vi "p2.vi"() -> ()   [LabVIEW 2021, in "d22.lvlib"]
uses:
  d22.lvlib
  AOC/AOC.lvlib
panel:
  out "Total Instructions":i32
  out "Instruction":i32
  out "Vis":T1(graph)
  out "facing":enum16{"R", "D", "L", "U"}(ring)=enum."L"
  out "col":i32=43
  out "row":i32=133
  in  "Example":string="        ...#\n        .#..\n        #...\n        ....\n...#.......#\n........#...\n..#....#....\n..........#.\n        ...#....\n        .....#..\n        .#......\n        ......#.\n\n10R5L5R10L4R5L5"
  in  "Example":bool
  out "Answer":i32=133174
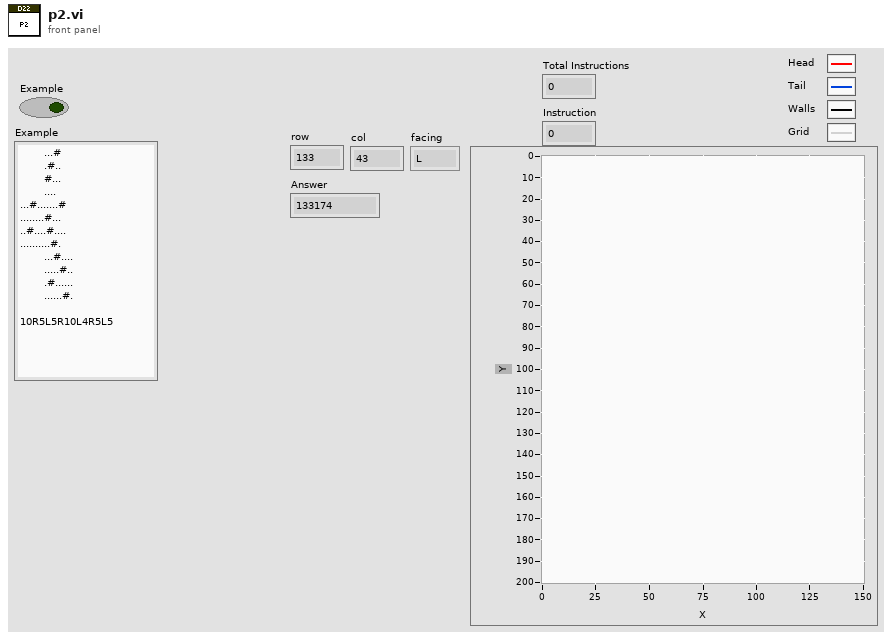
[diagram p1: front panel]
types:
  T1 = cluster{"index of element":i32[], "index of element":i32[]}[]
  T2 = cluster{"index of element":i32[], "index of element":i32[]}
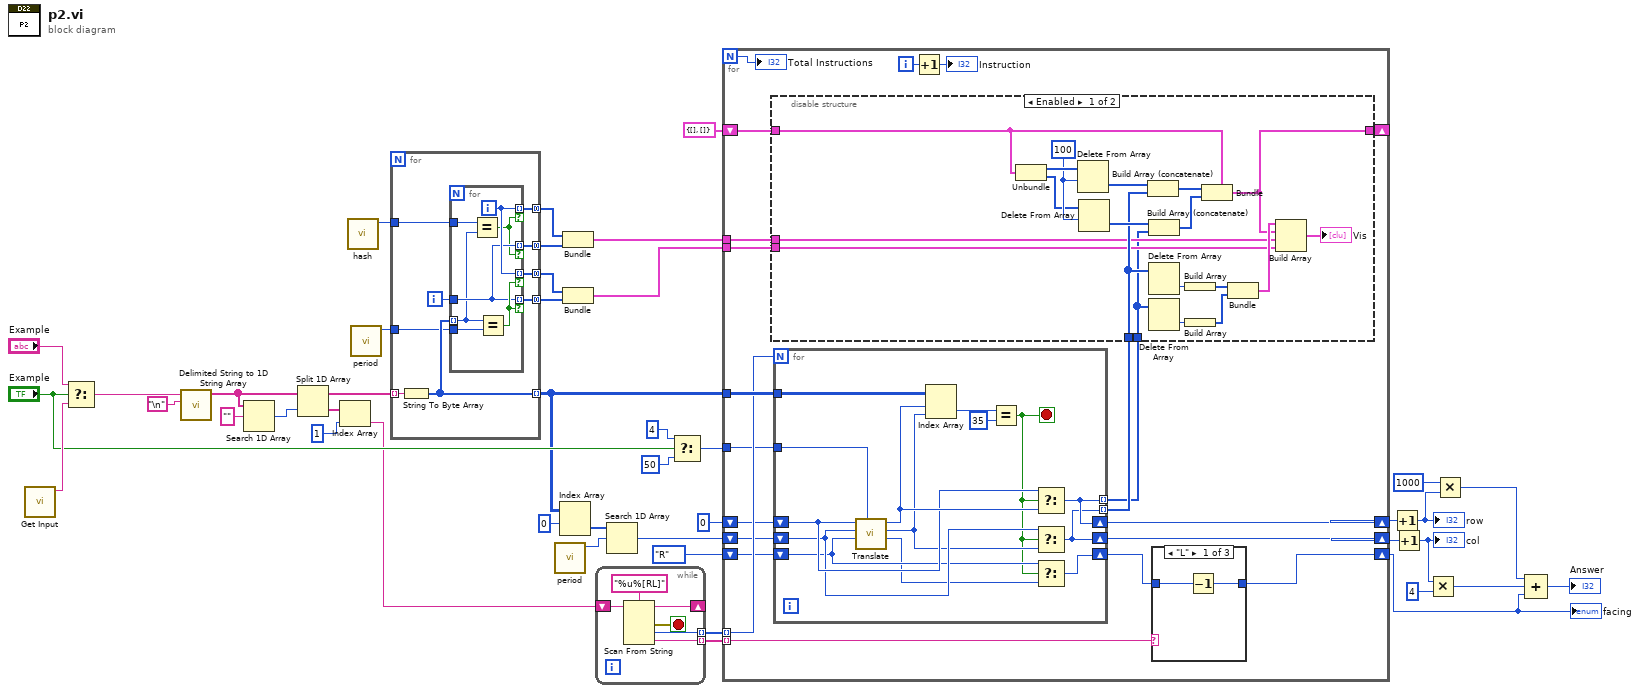
[diagram p0: block diagram]
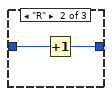
[diagram p3: hidden frame]
diagram:
  n1 = call "Get Input.vi"() -> ("Input"=w43:string)  [unwired: 11 in]
  n2 = Select(t="Example", s="Example", f=w43) -> (s? t:f=w42:string)
  n3 = call <vilib>:"Delimited String to 1D String Array.vi"("delimiter"="\n", "delimited string"=w42) -> ("string array"=w35:string[])  [unwired: 9 in]
  n4 = Search 1D Array(1D array=w35, element="") -> (index of element=w33:i32)  [unwired: 1 in]
  n5 = Split 1D Array(array=w35, index=w33) -> (first subarray=w34:string[], second subarray=w30:string[])
  n6 = Index Array(array=w30, index=1) -> (element=w28:string)
  n7 = call "hash.vi"() -> ("#"=w3:u8)  [unwired: 11 in]
  n8 = call "period.vi"() -> ("."=w7:u8)  [unwired: 11 in]
  n9 = for {
    tunnel: w34 -> [w52] mode=indexing
    tunnel: [w51] -> w23 mode=indexing
    tunnel: [w49] -> w10 mode=concatenating
    tunnel: [w48] -> w9 mode=concatenating
    tunnel: w7 -> [w47]
    tunnel: [w46] -> w6 mode=concatenating
    tunnel: [w45] -> w5 mode=concatenating
    tunnel: w3 -> [w44]
    i -> [w50]
    n10 = String To Byte Array(string=w52) -> (unsigned byte array=w51:u8[])
    n11 = for {
      tunnel: w51 -> [w55] mode=indexing
      tunnel: w50 -> [w56]
      tunnel: [w57] -> w49 mode=indexing if=w59
      tunnel: [w56] -> w48 mode=indexing if=w59
      tunnel: w47 -> [w58]
      tunnel: [w57] -> w46 mode=indexing if=w53
      tunnel: [w56] -> w45 mode=indexing if=w53
      tunnel: w44 -> [w54]
      i -> [w57]
      n12 = Equal?(x=w54, y=w55) -> (x = y?=w53:bool)
      n13 = Equal?(x=w55, y=w58) -> (x = y?=w59:bool)
    }
  }
  n14 = call "period.vi"() -> ("."=w24:u8)  [unwired: 11 in]
  n15 = Index Array(array=w23, index (row)=0) -> (element=w37:u8[])  [unwired: 1 in]
  n16 = Bundle(w6, w5) -> (w4:cluster{i32[], i32[]})  [unwired: 1 in]
  n17 = Bundle(w10, w9) -> (w8:cluster{i32[], i32[]})  [unwired: 1 in]
  n18 = while {
    shift-right: [w60] -> _
    shift-left: w28 -> [w65]
    tunnel: [w62] -> w26 mode=indexing
    tunnel: [w63] -> w27 mode=indexing
    stop <- w61 stop-if-true
    n19 = Scan From String(format string="%u%[RL]", input string=w65) -> (remaining string=w60:string, error out=w61:errorcluster, output 1=w63:u32, output 2=w62:string)  [unwired: 4 in, 1 out]
  }
  n20 = Search 1D Array(1D array=w37, element=w24) -> (index of element=w32:i32)  [unwired: 1 in]
  n21 = Select(t=4, s="Example", f=50) -> (s? t:f=w12:i32)
  n22 = for {
    N -> [w68]
    tunnel: w23 -> [w84]
    shift-right: [w81] -> w21
    shift-left: w32 -> [w74]
    shift-right: [w77] -> w22
    shift-left: 0 ("index of element") -> [w75]
    tunnel: w27 -> [w83] mode=indexing
    tunnel: w26 -> [w82] mode=indexing
    shift-right: [w85] -> w2
    shift-left: enum16{"R", "D", "L", "U"}."R" -> [w80]
    tunnel: w12 -> [w78]
    shift-right: [w72] -> _
    shift-left: T2 {"index of element"=[], "index of element"=[]} ("output cluster") -> [w76]
    tunnel: w8 -> [w70]
    tunnel: w4 -> [w71]
    i -> [w69]
    n23 = for {
      N: w83 -> [_]
      tunnel: w84 -> [w119]
      shift-right: [w106] -> w81
      shift-left: w74 -> [w111]
      shift-right: [w112] -> w77
      shift-left: w75 -> [w116]
      shift-right: [w115] -> w79
      shift-left: w80 -> [w109]
      tunnel: w78 -> [w114]
      tunnel: [w112] -> w66 mode=indexing
      tunnel: [w106] -> w73 mode=indexing
      stop <- w107 stop-if-true
      n24 = call "Translate.vi"("Size"=w114, "direction in"=w109, "x in"=w111, "y in"=w116) -> ("direction out"=w108:enum16{"R", "D", "L", "U"}, "x out"=w110:i32, "y out"=w117:i32)  [unwired: 5 in]
      n25 = Index Array(array=w119, index (row)=w117, index (col)=w110) -> (element=w113:u8)
      n26 = Equal?(x=w113, y=u8 35 ("x")) -> (x = y?=w107:bool)
      n27 = Select(t=w116, s=w107, f=w117) -> (s? t:f=w112:i32)
      n28 = Select(t=w111, s=w107, f=w110) -> (s? t:f=w106:i32)
      n29 = Select(t=w109, s=w107, f=w108) -> (s? t:f=w115:enum16{"R", "D", "L", "U"})
    }
    n30 = disable-structure shown="Enabled" {
      disable-tunnel: w76 -> [w104 w105]
      disable-tunnel: w73 -> [w96 _]
      disable-tunnel: [w90 w105] -> w72
      disable-tunnel: w71 -> [w89 _]
      disable-tunnel: w70 -> [w88 _]
      disable-tunnel: w66 -> [w87 _]
      frame Enabled {
        w98 = 100 ("length")
        n31 = Unbundle(w104) -> ("index of element"=w103:i32[], "index of element"=w86:i32[])
        n32 = Delete From Array(array=w103, length=w98) -> (deleted portion=w100:i32[])  [unwired: 1 in, 1 out]
        n33 = Delete From Array(array=w86, length=w98) -> (deleted portion=w99:i32[])  [unwired: 1 in, 1 out]
        n34 = Build Array (concatenate)(w100, w96) -> (w101:i32[])
        n35 = Build Array (concatenate)(w99, w87) -> (w102:i32[])
        n36 = Delete From Array(array=w96) -> (deleted portion=w95:i32)  [unwired: 2 in, 1 out]
        n37 = Delete From Array(array=w87) -> (deleted portion=w97:i32)  [unwired: 2 in, 1 out]
        n38 = Build Array(w95) -> (w93:i32[])
        n39 = Build Array(w97) -> (w94:i32[])
        n40 = Bundle(cluster=w104, "index of element"=w101, "index of element"=w102) -> (w90:T2)
        n41 = Bundle(w93, w94) -> (w92:cluster{i32[], i32[]})  [unwired: 1 in]
        n42 = Build Array(w92, w90, w89, w88) -> (→"Vis":T1)
      }
      frame Disabled {
      }
    }
    n43 = Increment(x=w69) -> (x+1=→"Instruction":i32)
    n44 = case shown="\"L\"" w82 {
      tunnel: [w120 w122 w124] -> w85
      tunnel: w79 -> [w121 w123 w124]
      frame "L" {
        n45 = Decrement(x=w121) -> (x-1=w120:enum16{"R", "D", "L", "U"})
      }
      frame "R" {
        n46 = Increment(x=w123) -> (x+1=w122:enum16{"R", "D", "L", "U"})
      }
      frame Default {
      }
    }
    "Total Instructions" <- w68
  }
  "facing" <- w2
  n47 = Increment(x=w22) -> (x+1=w20:i32)
  "row" <- w20
  n48 = Increment(x=w21) -> (x+1=w18:i32)
  "col" <- w18
  n49 = Multiply(x=w18, y=4 ("x+1")) -> (x*y=w15:i32)
  n50 = Multiply(x=1000, y=w20) -> (x*y=w16:i32)
  n51 = Compound Arithmetic op=ADD(w16, w15, w2) -> (→"Answer":i32)
